vi "Post Tweet.vi"(8 "error in (no error)":errorcluster, 10 "Tweet":string, 11 "Twitter Handle In":T1={"OAuth Credentials"={"Consumer Key"="", "Signature Method"=enum."HMAC-SHA1", "Token"="", "Version"="", "Token Secret"="", "Consumer Secret"=""}, "since ID"="", "max ID"="", "Screen Name"=""}) -> (0 "error out":errorcluster, 3 "Twitter Handle Out":T1={"OAuth Credentials"={"Consumer Key"="", "Signature Method"=enum."HMAC-SHA1", "Token"="", "Version"="", "Token Secret"="", "Consumer Secret"=""}, "since ID"="", "max ID"="", "Screen Name"=""})   [LabVIEW 2011, in "i3-twitter.lvlib"]
doc: "Post status for the authenticting user."
uses:
  i3-twitter.lvlib
  Controls/Twitter Handle.ctl
  i3-oauth/Controls/OAuth Credentials.ctl
  i3-oauth/Controls/Signature Method.ctl
  i3-oauth/Controls/HTTP Method.ctl
  <vilib>/httpClient/POSTBuffer.vi
  i3-oauth/i3-oauth.lvlib
  <vilib>/httpClient/LabVIEWHTTPClient.lvlib
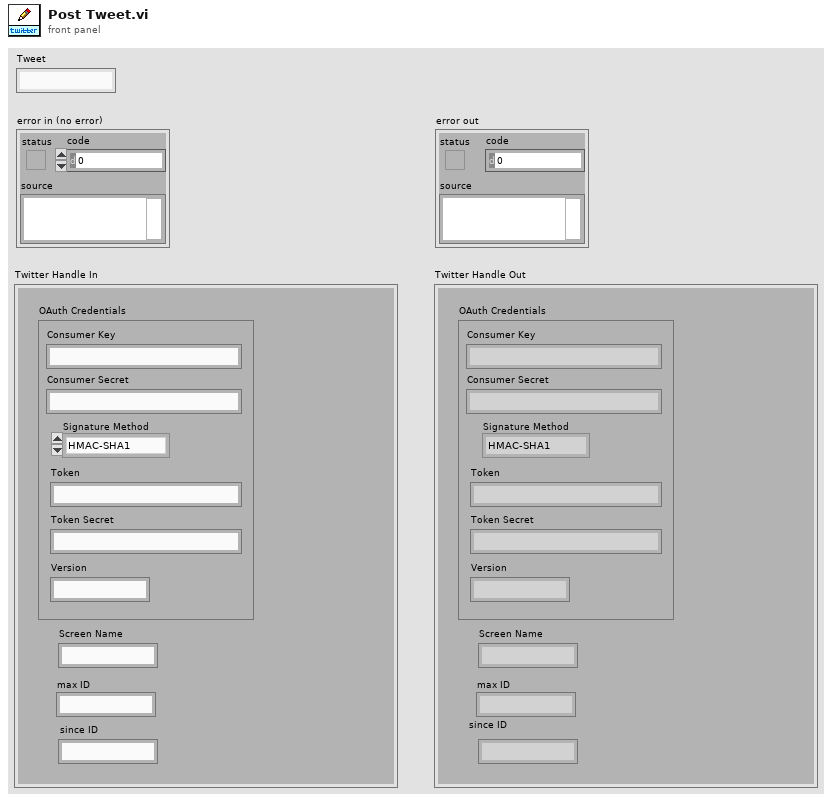
[diagram p1: front panel]
types:
  T1 = typedef "i3-twitter.lvlib/Twitter Handle.ctl" = cluster{"OAuth Credentials":T2, "since ID":string, "max ID":string, "Screen Name":string}
  T2 = typedef "i3-oauth.lvlib/OAuth Credentials.ctl" = cluster{"Consumer Key":string, "Signature Method":T3, "Token":string, "Version":string, "Token Secret":string, "Consumer Secret":string}
  T3 = typedef "i3-oauth.lvlib/Signature Method.ctl" = enum16{"HMAC-MD5", "HMAC-SHA1", "HMAC-SHA224", "HMAC-SHA256", "HMAC-SHA384", "HMAC-SHA512"}
  T4 = typedef "i3-oauth.lvlib/HTTP Method.ctl" = enum16{"GET", "POST", "PUT", "DELETE"}
  T5 = typedef "i3-oauth.lvlib/key-value-pairs.ctl" = cluster{"key":string, "value":string}
  T6 = typedef "LabVIEWHTTPClient.lvlib/ClientHandle.ctl" = refnum<k1>
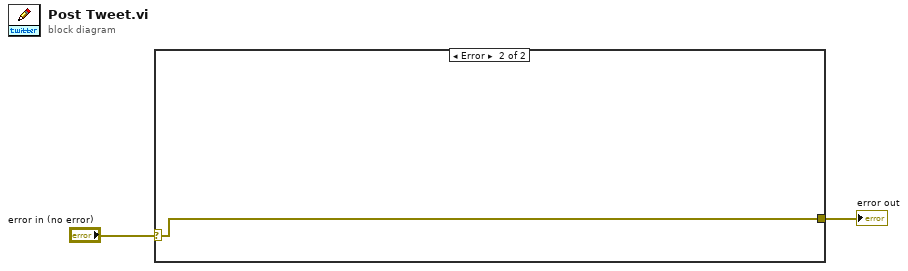
[diagram p0: block diagram]
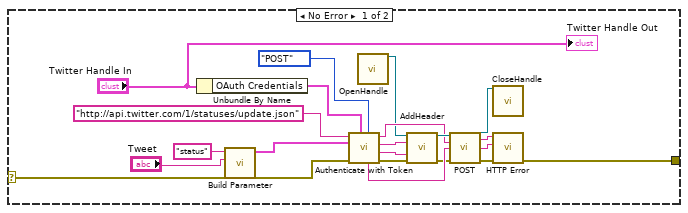
[diagram p2: hidden frame]
diagram:
  n1 = case shown="Error" "error in (no error)" {
    selector: "error in (no error)" -> [w3 w24]
    tunnel: [w8 w24] -> w2
    frame No Error {
      n2 = Unbundle By Name("Twitter Handle In") -> ("OAuth Credentials"=w12:T2)
      n3 = call "Build Parameter.vi"("Value"="Tweet", "Key"="status") -> ("Parameter Array"=w14:T5[])  [unwired: 9 in]
      n4 = call "Authenticate with Token.vi"("HTTP Method"=HTTP_Method."POST", "Body Parameters"=w14, "OAuth Credentials"=w12, "error in (no error)"=w3, "Base URL"="http://api.twitter.com/1/statuses/update.json") -> ("error out"=w5:errorcluster, "Header Value"=w19:string, "Header Parameter"=w18:string, "Full URL"=w15:string, "Body"=w16:string)  [unwired: 2 in]
      n5 = call <vilib>:"OpenHandle.vi"() -> ("client handle out"=w7:T6)  [unwired: 14 in, 1 out]
      n6 = call <vilib>:"AddHeader.vi"("client handle"=w7, "header"=w18, "value"=w19, "error in (no error)"=w5) -> ("client handle out"=w17:T6, "error out"=w4:errorcluster)  [unwired: 10 in]
      n7 = call-poly <vilib>:"POST.vi"("client handle"=w17, "url"=w15, "data"=w16, "error in (no error)"=w4) -> ("client handle out"=w6:T6, "headers"=w11:string, "body"=w10:string, "error out"=w9:errorcluster)  [unwired: 8 in]
      n8 = call <vilib>:"CloseHandle.vi"("client handle"=w6) -> ()  [unwired: 14 in, 1 out]
      n9 = call "HTTP Error.vi"("error in (no error)"=w9, "Body"=w10, "Header"=w11) -> ("error out"=w8:errorcluster)  [unwired: 6 in, 2 out]
      "Twitter Handle Out" <- "Twitter Handle In"
    }
    frame Error {
    }
  }
  "error out" <- w2
